vi "CoordsToPath.vi"(8 "error in (no error)":errorcluster, 10 "Coords":T1, 11 "CtlRef":refnum<vi>) -> (0 "error out":errorcluster, 2 "Item Path":string)   [LabVIEW 2013]
uses:
  <vilib>/Utility/miscctls.llb/LVPoint32TypeDef.ctl
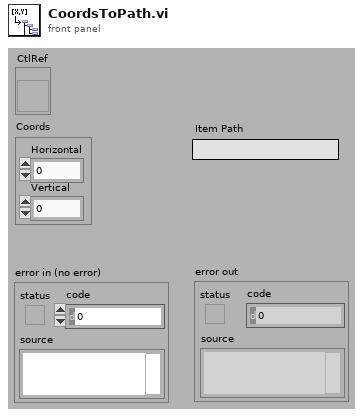
[diagram p1: front panel]
types:
  T1 = typedef "LVPoint32TypeDef.ctl" = cluster{"Horizontal":i32, "Vertical":i32}
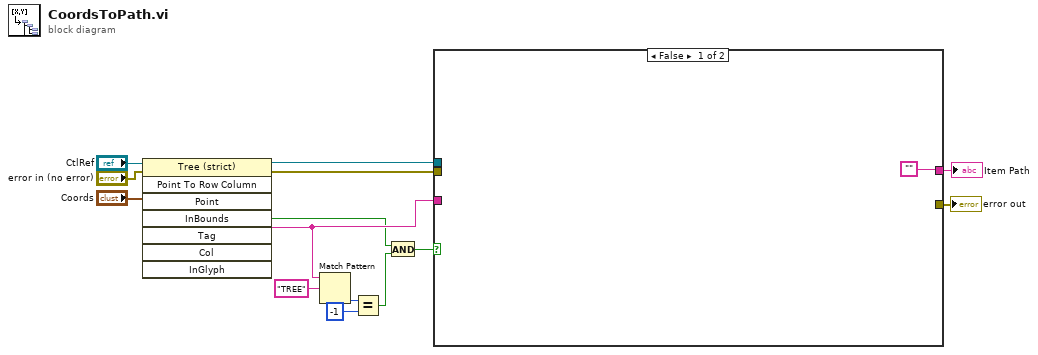
[diagram p0: block diagram]
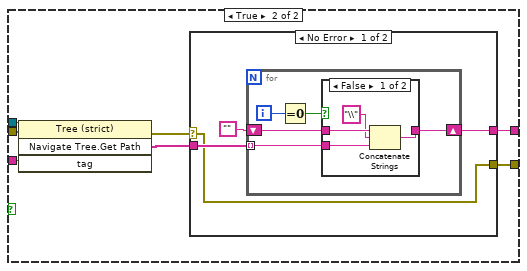
[diagram p2: hidden frame]
diagram:
  n1 = invoke class="Tree (strict)" method="Point To Row Column"(reference="CtlRef", error in="error in (no error)", "Point"="Coords") -> (reference out=w13:refnum<vi>, error out=w14:errorcluster, "InBounds"=w2:bool, "Tag"=w7:string)  [unwired: 5 in, 4 out]
  n2 = Match Pattern(string=w7, regular expression="TREE") -> (offset past match=w5:i32)  [unwired: 1 in, 3 out]
  n3 = Equal?(x=w5, y=-1) -> (x = y?=w3:bool)
  n4 = And(x=w2, y=w3) -> (x .and. y?=w1:bool)
  n5 = case shown="False" w1 {
    tunnel: w14 -> [_ w22]
    tunnel: w13 -> [_ w21]
    tunnel: ["" w20] -> w10
    tunnel: [_ w17] -> w8
    tunnel: w7 -> [_ w16]
    frame False {
    }
    frame True {
      n6 = invoke class="Tree (strict)" method="Navigate Tree.Get Path"(reference=w21, error in=w22, "tag"=w16) -> (error out=w18:errorcluster, "Navigate Tree:Get Path"=w19:string[])  [unwired: 1 in, 2 out]
      n7 = case shown="No Error" w18 {
        selector: w18 -> [w23 _]
        tunnel: [w25 _] -> w20
        tunnel: w19 -> [w24 _]
        tunnel: [w23 _] -> w17
        frame No Error {
          n8 = for {
            shift-right: [w28] -> w25
            shift-left: "" -> [w27]
            tunnel: w24 -> [w29] mode=indexing
            i -> [w31]
            n9 = Equal To 0?(x=w31) -> (x = 0?=w30:bool)
            n10 = case shown="False" w30 {
              tunnel: w29 -> [w32 w36]
              tunnel: [w35 w36] -> w28
              tunnel: w27 -> [w34 _]
              frame False {
                n11 = Concatenate Strings(w34, "\\" ("string"), w32) -> (w35:string)
              }
              frame True {
              }
            }
          }
        }
        frame Error {
        }
      }
    }
  }
  "error out" <- w8
  "Item Path" <- w10
